vi "Determine Warnings(Challenge).vi"() -> ()   [LabVIEW 2014]
panel:
  out "Warning?":bool
  out "Warning Text":string
  in  "Min Temp 2":dbl
  in  "Max Temp":dbl
  in  "Current Temp":dbl
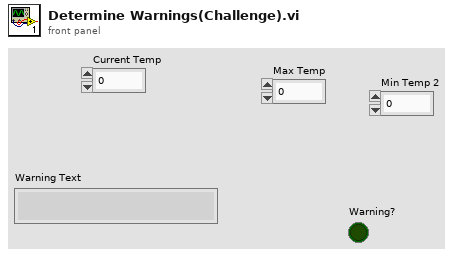
[diagram p1: front panel]
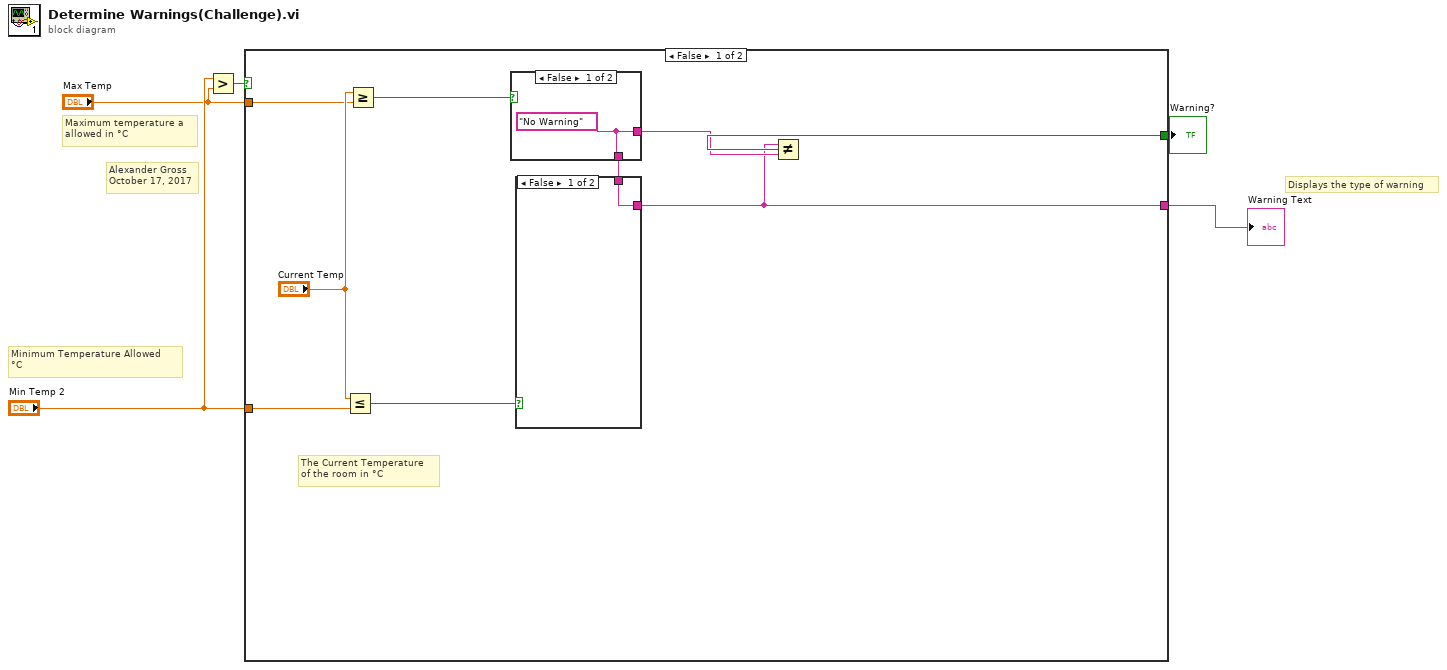
[diagram p0: block diagram]
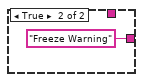
[diagram p2: hidden frame]
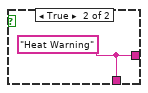
[diagram p3: hidden frame]
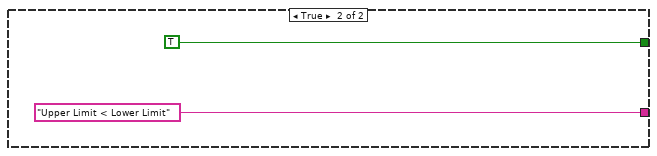
[diagram p4: hidden frame]
diagram:
  # "Alexander Gross\nOctober 17, 2017"
  # "Displays the type of warning"
  # "Minimum Temperature Allowed\n°C"
  # "Maximum temperature a\nallowed in °C"
  n1 = Greater?(x="Min Temp 2", y="Max Temp") -> (0:w1:bool)
  n2 = case shown="False" w1 {
    tunnel: [w7 "Upper Limit < Lower Limit"] -> w5
    tunnel: [w13 TRUE] -> w4
    tunnel: "Min Temp 2" -> [w12 _]
    tunnel: "Max Temp" -> [w11 _]
    frame False {
      # "The Current Temperature \nof the room in °C"
      n3 = Less Or Equal?(x="Current Temp", y=w12) -> (x <= y?=w9:bool)
      n4 = Greater Or Equal?(x="Current Temp", y=w11) -> (x >= y?=w10:bool)
      n5 = case shown="False" w10 {
        tunnel: [w17 w18] -> w8
        tunnel: [w17 w18] -> w6
        frame False {
          w17 = "No Warning"
        }
        frame True {
          w18 = "Heat Warning"
        }
      }
      n6 = case shown="False" w9 {
        tunnel: [w15 "Freeze Warning"] -> w7
        tunnel: w6 -> [w15 _]
        frame False {
        }
        frame True {
        }
      }
      n7 = Not Equal?(x=w7, y=w8) -> (x != y?=w13:bool)
    }
    frame True {
    }
  }
  "Warning Text" <- w5
  "Warning?" <- w4
